vi "CTRE_Phoenix_CANdle_ModulateVBatOutput.vi"(0 "CTRE_CANdle_DeviceRef":T1, 5 "Duty Cycle Percent":dbl min=0.0 max=1.0 step=0.0001, 11 "error in":errorcluster) -> (4 "CTRE_CANdle_DeviceRef":T1, 15 "error out":errorcluster)   [LabVIEW 2020]
doc: "Modulates the VBat output to the specified duty cycle percentage.\n\nThis VI will only take effect if the VBatOutput config is set to \"Modulated\".\n\n<b>Duty Cycle Percent</b> is the percent duty cycle from 0 to 1"
uses:
  <vilib>/Rock Robotics/WPI/ThirdParty/Phoenix-LabVIEW/CANdle/Controls/CTRE_Phoenix_CANdle_DeviceRef.ctl
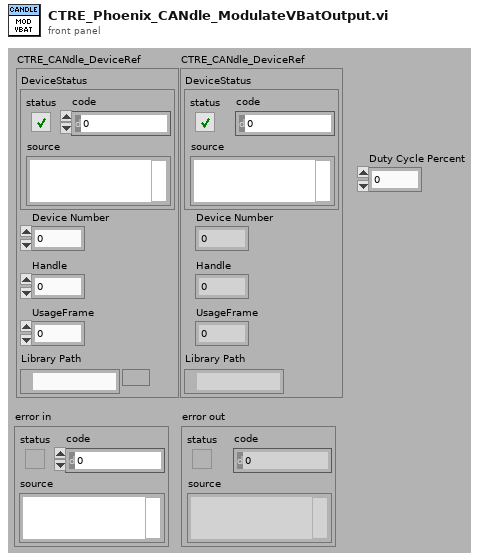
[diagram p1: front panel]
types:
  T1 = typedef "CTRE_Phoenix_CANdle_DeviceRef.ctl" = cluster{"DeviceStatus":errorcluster, "Device Number":u8, "Handle":u64, "UsageFrame":u32, "Library Path":path}
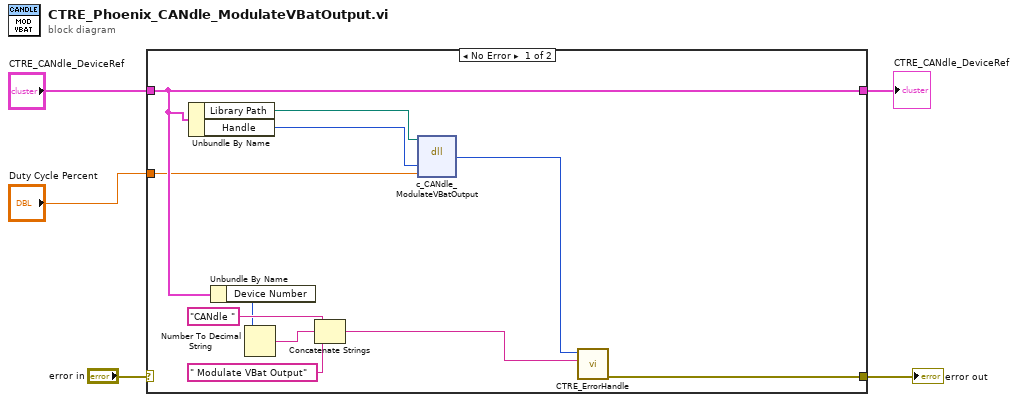
[diagram p0: block diagram]
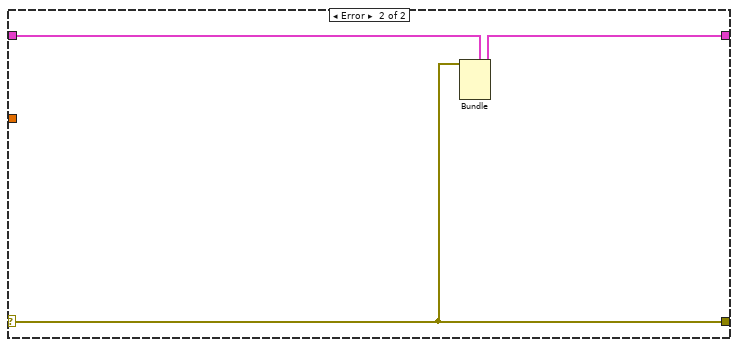
[diagram p2: hidden frame]
diagram:
  n1 = case shown="No Error" "error in" {
    selector: "error in" -> [_ w18]
    tunnel: "CTRE_CANdle_DeviceRef" -> [w9 w19]
    tunnel: [w16 w18] -> w5
    tunnel: [w9 w17] -> w2
    tunnel: "Duty Cycle Percent" -> [w6 _]
    frame No Error {
      n2 = Unbundle By Name(w9) -> ("Library Path"=w8:path, "Handle"=w7:u64)
      n3 = Unbundle By Name(w9) -> ("Device Number"=w12:u8)
      n4 = Number To Decimal String(number=w12) -> (decimal integer string=w14:string)  [unwired: 1 in]
      n5 = Concatenate Strings("CANdle " ("string"), w14, " Modulate VBat Output" ("string")) -> (w10:string)
      n6 = dll-call lib="?" fn="c_CANdle_ModulateVBatOutput"(path in=w8, "handle"=w7, "dutyCyclePercent"=w6) -> ("return type"=w11:i32)  [unwired: 4 in, 2 out]
      n7 = call <vilib>:"CTRE_ErrorHandle.vi"("origin"=w10, "code"=w11) -> ("error out"=w16:errorcluster)  [unwired: 9 in]
    }
    frame Error {
      n8 = Bundle(cluster=w19, "DeviceStatus"=w18) -> (w17:T1)  [unwired: 4 in]
    }
  }
  "error out" <- w5
  "CTRE_CANdle_DeviceRef" <- w2
